vi "Detect.vi"(5 "server-ip":string, 6 "client-ip":string, 7 "dut-ip":string) -> (2 "dut-mac":string, 3 "布尔":bool=TRUE)   [LabVIEW 2014]
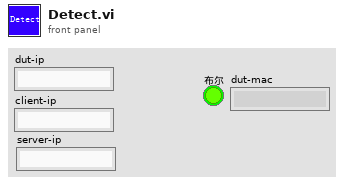
[diagram p1: front panel]
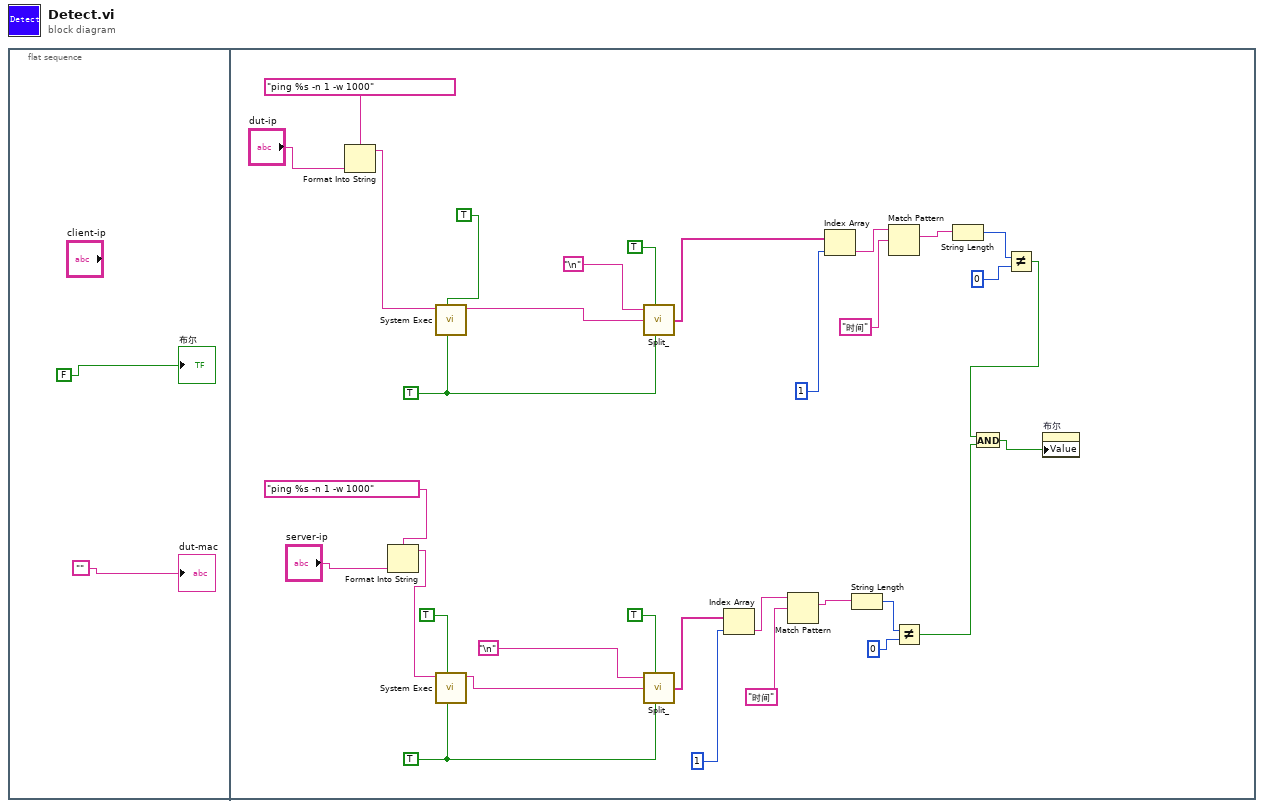
[diagram p0: block diagram]
diagram:
  n1 = flat-sequence {
    frame #0 {
      "布尔" <- FALSE
      "dut-mac" <- ""
    }
    frame #1 {
      w19 = TRUE
      w33 = TRUE
      n2 = Format Into String(format string="ping %s -n 1 -w 1000", "dut-ip") -> (resulting string=w4:string)  [unwired: 2 in, 1 out]
      n3 = Format Into String(format string="ping %s -n 1 -w 1000", "server-ip") -> (resulting string=w21:string)  [unwired: 2 in, 1 out]
      n4 = call <vilib>:"System Exec.vi"("run minimized? (F)"=w33, "wait until completion? (T)"=TRUE, "command line"=w4) -> ("standard output"=w3:string)  [unwired: 5 in, 3 out]
      n5 = call <vilib>:"System Exec.vi"("run minimized? (F)"=w19, "wait until completion? (T)"=TRUE, "command line"=w21) -> ("standard output"=w18:string)  [unwired: 5 in, 3 out]
      n6 = call "Split_.vi"("分隔字符串/字符(,)"="\n", "移除空字符串（T）"=TRUE, "字符串"=w3, "移除空白字符（T）"=w33) -> ("字符串数组"=w30:string[])  [unwired: 3 in]
      n7 = call "Split_.vi"("分隔字符串/字符(,)"="\n", "移除空字符串（T）"=TRUE, "字符串"=w18, "移除空白字符（T）"=w19) -> ("字符串数组"=w15:string[])  [unwired: 3 in]
      n8 = Index Array(array=w15, index=1) -> (element=w13:string)
      n9 = Match Pattern(string=w13, regular expression="时间") -> (match substring=w11:string)  [unwired: 1 in, 3 out]
      n10 = Index Array(array=w30, index=1) -> (element=w28:string)
      n11 = String Length(string=w11) -> (length=w9:i32)
      n12 = Match Pattern(string=w28, regular expression="时间") -> (match substring=w26:string)  [unwired: 1 in, 3 out]
      n13 = Not Equal?(x=w9, y=0) -> (x != y?=w6:bool)
      n14 = String Length(string=w26) -> (length=w24:i32)
      n15 = Not Equal?(x=w24, y=0) -> (x != y?=w7:bool)
      n16 = And(x=w7, y=w6) -> (x .and. y?=w5:bool)
      n17 = property on="布尔" class="Bool (严格)"("Value"=w5) -> ()  [unwired: 2 in, 2 out]
    }
  }
